vi "Get Buffer Size in Bytes.vi"(8 "error in (no error)":errorcluster, 11 "Buffer Data in":refnum<class "Buffer.lvclass">) -> (0 "error out":errorcluster, 2 "Buffer Size (bytes)":i32, 3 "Buffer Data":refnum<class "Buffer.lvclass">)   [LabVIEW 2020, in "Buffer.lvclass"]
uses:
  Buffer.lvclass
  Buffer.lvclass/Buffer.ctl
  <vilib>/Utility/error.llb/Error Cluster From Error Code.vi
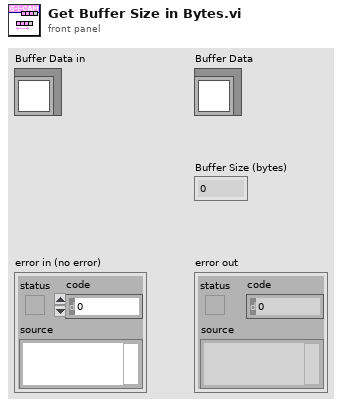
[diagram p1: front panel]
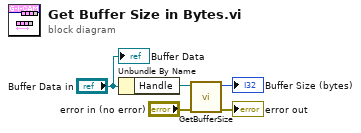
[diagram p0: block diagram]
diagram:
  n1 = Unbundle By Name("Buffer Data in") -> ("Handle"=w2:refnum<data-value>)
  n2 = call "GetBufferSize.vi"("error in (no error)"="error in (no error)", "Handle"=w2) -> ("error out"=→"error out":errorcluster, "Size"=→"Buffer Size (bytes)":i32)  [unwired: 8 in]
  "Buffer Data" <- "Buffer Data in"
